vi "truncate 2D array double.vi"(2 "b-t-l-r":i32[](array[numeric]), 3 "Array in":dbl[][](array[numeric])) -> (1 "Array out":dbl[][](array[numeric]))   [LabVIEW 2018]
panel:
  # "bottom"
  # "top"
  # "left"
  # "right"
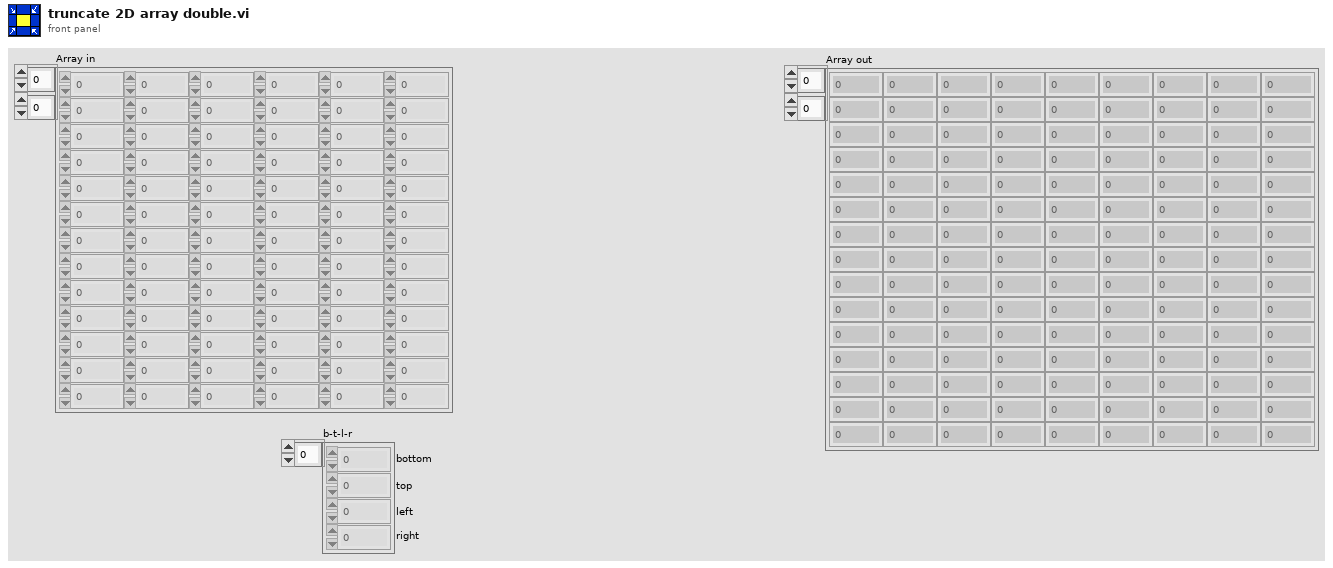
[diagram p1: front panel]
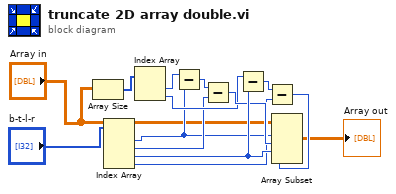
[diagram p0: block diagram]
diagram:
  n1 = Array Size(array="Array in") -> (size(s)=w4:i32[])
  n2 = Index Array(array="b-t-l-r") -> (element #1=w6:i32, element #2=w8:i32, element #3=w14:i32, element #4=w11:i32)  [unwired: 4 in]
  n3 = Index Array(array=w4) -> (element #1=w5:i32, element #2=w10:i32)  [unwired: 2 in]
  n4 = Subtract(x=w5, y=w6) -> (x-y=w7:i32)
  n5 = Subtract(x=w7, y=w8) -> (x-y=w12:i32)
  n6 = Subtract(x=w10, y=w14) -> (x-y=w9:i32)
  n7 = Subtract(x=w9, y=w11) -> (x-y=w13:i32)
  n8 = Array Subset(array="Array in", index (row)=w6, length (row)=w12, index (col)=w14, length (col)=w13) -> (→"Array out":dbl[][])
